vi "Update Staff Allocation.vi"(0 "File Data Manager in":refnum<class "File Data Manager.lvclass">, 5 "Staff Name":string[](array[string]), 7 "Service ID":string[](array[string]), 11 "error in (no error)":errorcluster) -> (4 "File Data Manager out":refnum<class "File Data Manager.lvclass">, 15 "error out":errorcluster)   [LabVIEW 2023, in "File Data Manager.lvlib" / "File Data Manager.lvclass"]
uses:
  File Data Manager.lvclass
  File Data Manager.lvclass/File Data Manager.ctl
  <vilib>/Utility/miscctls.llb/LVMapReplaceAction.ctl
  <vilib>/ActorFramework/Actor/Actor.lvclass
  Central Data Manager/Central Data Manager Messages/Refresh Rooms Status Msg/Refresh Rooms Status Msg.lvclass
  C:/Users/bhaghyaraj/Trainings/NI Actor Framework/SDLC/Central Data Manager/Central Data Manager/Central Data Manager.lvclass
  C:/Users/bhaghyaraj/Trainings/NI Actor Framework/SDLC/Model Base/Model Base/Model Base.lvclass
  C:/Program Files/National Instruments/LabVIEW 2023/vi.lib/ActorFramework/Actor/Actor.lvclass
  C:/Users/bhaghyaraj/Trainings/NI Actor Framework/SDLC/Interfaces/Model Base/Incoming Model Base Interface.lvclass
  C:/Users/bhaghyaraj/Trainings/NI Actor Framework/SDLC/File Data Manager/File Data Manager/File Data Manager.lvclass
  Room Service Types/Room Service Base/Room Service Base.lvclass
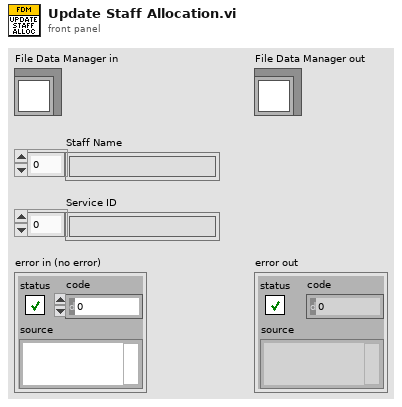
[diagram p1: front panel]
types:
  T1 = map{string, map{string, refnum<class "Room Service Base.lvclass">}}
  T2 = map{string, refnum<class "Room Service Base.lvclass">}
  T3 = typedef "LVMapReplaceAction.ctl" = enum32{"Modify Entry only if found", "Add or Modify Entry", "Delete Entry"}
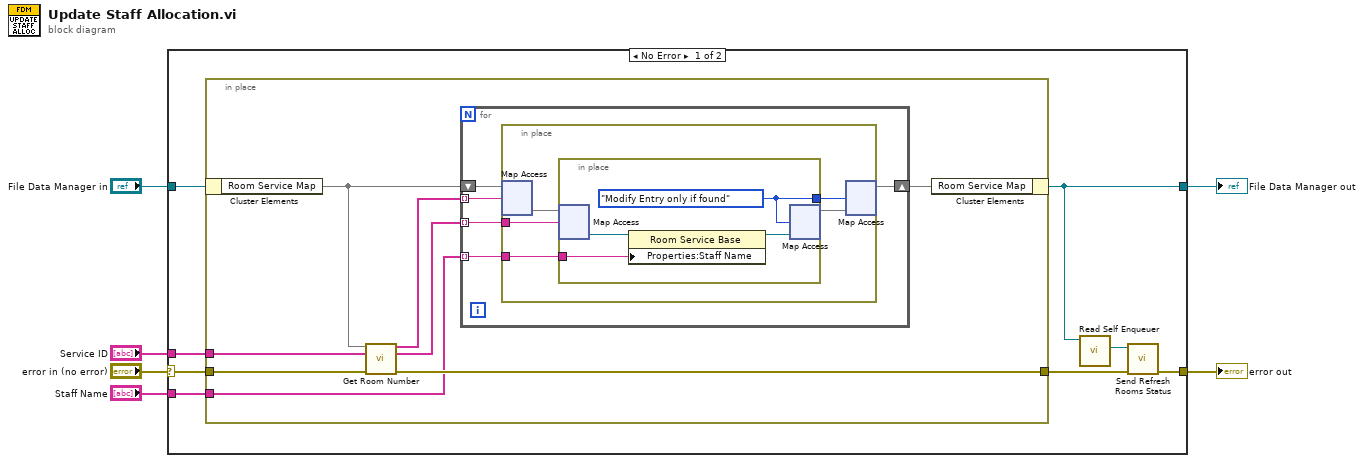
[diagram p0: block diagram]
diagram:
  n1 = case shown="No Error" "error in (no error)" {
    selector: "error in (no error)" -> [w13 w37]
    tunnel: [w9 w37] -> w4
    tunnel: "File Data Manager in" -> [w11 w38]
    tunnel: [w10 w38] -> w3
    tunnel: "Service ID" -> [w14 _]
    tunnel: "Staff Name" -> [w7 _]
    frame No Error {
      n2 = in-place {
        in-place-border: w14 -> [w22]
        in-place-border: w13 -> [w21]
        in-place-border: [w20] -> w12
        in-place-border: w7 -> [w15]
        n3 = in-place-cluster #1(w11) -> ("Room Service Map"=w19:T1)
        n4 = call "Get Room Number.vi"("Room Service Map"=w19, "Service ID"=w22, "error in (no error)"=w21) -> ("Room Number"=w18:string[], "Service ID"=w17:string[], "error out"=w20:errorcluster)  [unwired: 10 in]
        n5 = for {
          shift-right: [w26] -> w16
          shift-left: w19 -> [w27]
          tunnel: w18 -> [w25] mode=indexing
          tunnel: w17 -> [w24] mode=indexing
          tunnel: w15 -> [w23] mode=indexing
          n6 = in-place {
            in-place-border: w24 -> [w30]
            in-place-border: w23 -> [w28]
            n7 = in-place-map #2(w27, w25) -> (w32:T2)  [unwired: 1 in, 1 out]
            n8 = in-place {
              in-place-border: [w35] -> w29
              in-place-border: w28 -> [w33]
              w35 = LVMapReplaceAction."Modify Entry only if found" ("action")
              n9 = in-place-map #3(w32, w30) -> (w34:refnum<class "Room Service Base.lvclass">)  [unwired: 1 in, 1 out]
              n10 = property class="Room Service Base"(reference=w34, "Properties:Staff Name"=w33) -> (reference out=w36:refnum<class "Room Service Base.lvclass">)  [unwired: 1 in, 1 out]
              n11 = in-place-map #3(w36, w35) -> (w31:T2)  [unwired: 2 out]
            }
            n12 = in-place-map #2(w31, w29) -> (w26:T1)  [unwired: 2 out]
          }
        }
        n13 = in-place-cluster #1("Room Service Map"=w16) -> (w10:refnum<class "File Data Manager.lvclass">)
      }
      n14 = call <vilib>:"Read Self Enqueuer.vi"("Actor"=w10) -> ("Self Enqueuer"=w8:refnum<class "Message Enqueuer.lvclass">)  [unwired: 10 in]
      n15 = call "Send Refresh Rooms Status.vi"("error in (no error)"=w12, "Message Enqueuer"=w8) -> ("error out"=w9:errorcluster)  [unwired: 8 in, 1 out]
    }
    frame Error {
    }
  }
  "error out" <- w4
  "File Data Manager out" <- w3
